vi "RTS Open TDMS Asycronous.vi"(6 "Tree Selection":T1, 7 "Debug":bool, 8 "Error In":errorcluster, 11 "TDMS Data Save Input":T2) -> (0 "Error Out":errorcluster, 3 "TDMS Data Save Output":T2)   [LabVIEW 2016]
uses:
  Type Definitions/RTS TDMS Filename Locations.ctl
  Type Definitions/RTS Room Selector.ctl
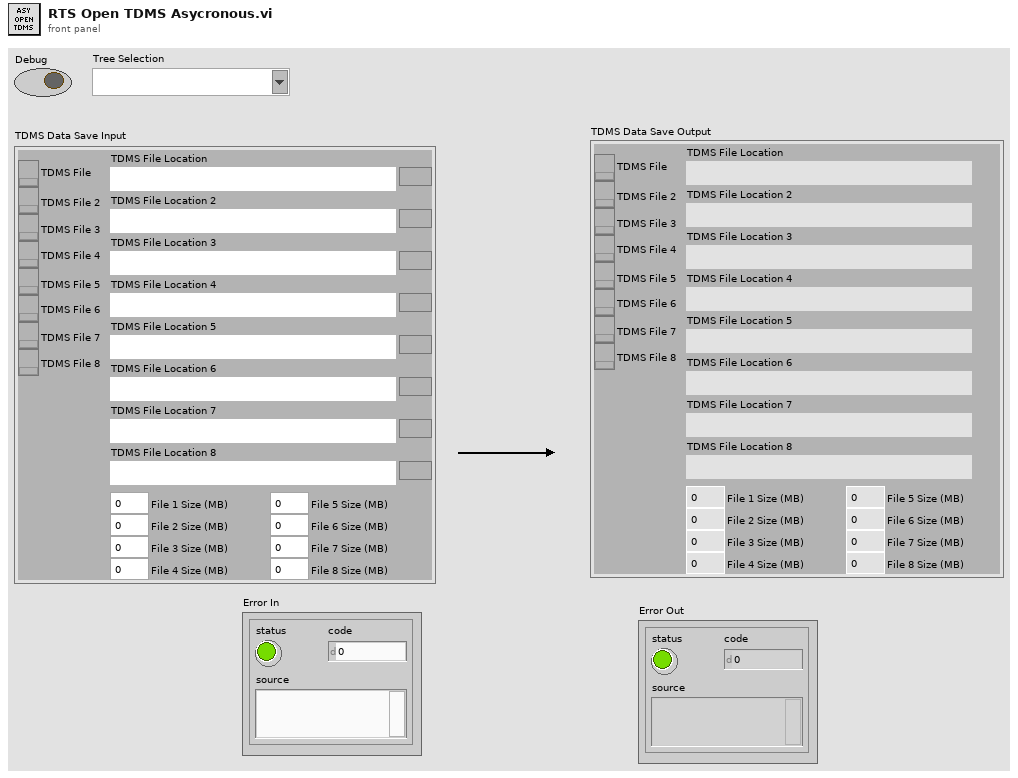
[diagram p1: front panel]
types:
  T1 = typedef "RTS Room Selector.ctl" = string
  T2 = typedef "RTS TDMS Filename Locations.ctl" = cluster{"TDMS File":refnum<k34>, "TDMS File Location":path, "TDMS File Location 2":path, "TDMS File Location 3":path, "TDMS File Location 4":path, "TDMS File Location 5":path, "TDMS File Location 6":path, "TDMS File Location 7":path, "TDMS File Location 8":path, "TDMS File 2":refnum<k34>, "TDMS File 3":refnum<k34>, "TDMS File 4":refnum<k34>, "TDMS File 5":refnum<k34>, "TDMS File 6":refnum<k34>, "TDMS File 7":refnum<k34>, "TDMS File 8":refnum<k34>, "File 1 Size (MB)":dbl, "File 2 Size (MB)":dbl, "File 3 Size (MB)":dbl, "File 4 Size (MB)":dbl, "File 5 Size (MB)":dbl, "File 6 Size (MB)":dbl, "File 7 Size (MB)":dbl, "File 8 Size (MB)":dbl}
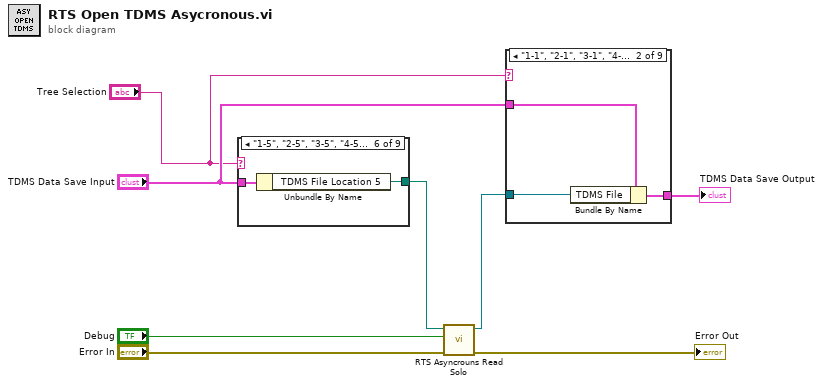
[diagram p0: block diagram]
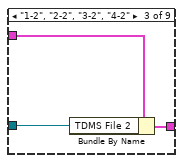
[diagram p3: hidden frame]
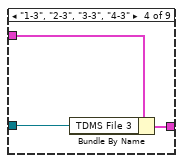
[diagram p4: hidden frame]
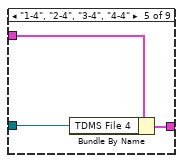
[diagram p5: hidden frame]
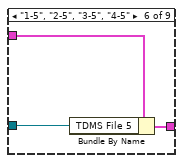
[diagram p6: hidden frame]
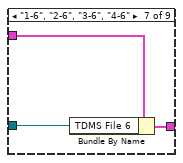
[diagram p7: hidden frame]
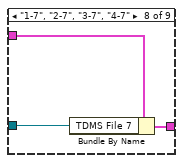
[diagram p8: hidden frame]
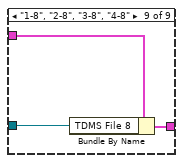
[diagram p9: hidden frame]
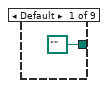
[diagram p10: hidden frame]
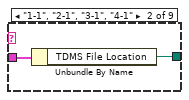
[diagram p11: hidden frame]
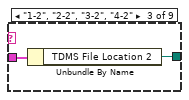
[diagram p12: hidden frame]
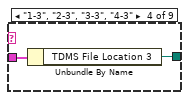
[diagram p13: hidden frame]
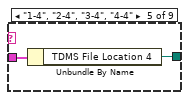
[diagram p14: hidden frame]
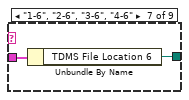
[diagram p15: hidden frame]
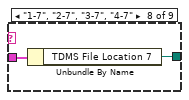
[diagram p16: hidden frame]
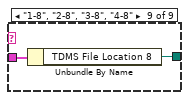
[diagram p17: hidden frame]
diagram:
  n1 = case shown="\"1-5\", \"2-5\", \"3-5\", \"4-5\"" "Tree Selection" {
    tunnel: "TDMS Data Save Input" -> [_ w11 w13 w15 w17 w19 w21 w23 w25]
    tunnel: [path "" ("TDMS File Location 8") w10 w12 w14 w16 w18 w20 w22 w24] -> w6
    frame Default {
    }
    frame "1-1", "2-1", "3-1", "4-1" {
      n2 = Unbundle By Name(w11) -> ("TDMS File Location"=w10:path)
    }
    frame "1-2", "2-2", "3-2", "4-2" {
      n3 = Unbundle By Name(w13) -> ("TDMS File Location 2"=w12:path)
    }
    frame "1-3", "2-3", "3-3", "4-3" {
      n4 = Unbundle By Name(w15) -> ("TDMS File Location 3"=w14:path)
    }
    frame "1-4", "2-4", "3-4", "4-4" {
      n5 = Unbundle By Name(w17) -> ("TDMS File Location 4"=w16:path)
    }
    frame "1-5", "2-5", "3-5", "4-5" {
      n6 = Unbundle By Name(w19) -> ("TDMS File Location 5"=w18:path)
    }
    frame "1-6", "2-6", "3-6", "4-6" {
      n7 = Unbundle By Name(w21) -> ("TDMS File Location 6"=w20:path)
    }
    frame "1-7", "2-7", "3-7", "4-7" {
      n8 = Unbundle By Name(w23) -> ("TDMS File Location 7"=w22:path)
    }
    frame "1-8", "2-8", "3-8", "4-8" {
      n9 = Unbundle By Name(w25) -> ("TDMS File Location 8"=w24:path)
    }
  }
  n10 = call "RTS Asyncrouns Read Solo.vi"("error in (no error)"="Error In", "Debug"="Debug", "TDMS File Location 8"=w6) -> ("error out"=→"Error Out":errorcluster, "Refnum out"=w4:refnum<k34>)  [unwired: 7 in]
  n11 = case shown="\"1-1\", \"2-1\", \"3-1\", \"4-1\"" "Tree Selection" {
    tunnel: "TDMS Data Save Input" -> [w26 w29 w32 w35 w38 w41 w44 w47 w50]
    tunnel: w4 -> [_ w27 w30 w33 w37 w39 w42 w45 w48]
    tunnel: [w26 w28 w31 w34 w36 w40 w43 w46 w49] -> w3
    frame Default {
    }
    frame "1-1", "2-1", "3-1", "4-1" {
      n12 = Bundle By Name(cluster=w29, "TDMS File"=w27) -> (w28:T2)
    }
    frame "1-2", "2-2", "3-2", "4-2" {
      n13 = Bundle By Name(cluster=w32, "TDMS File 2"=w30) -> (w31:T2)
    }
    frame "1-3", "2-3", "3-3", "4-3" {
      n14 = Bundle By Name(cluster=w35, "TDMS File 3"=w33) -> (w34:T2)
    }
    frame "1-4", "2-4", "3-4", "4-4" {
      n15 = Bundle By Name(cluster=w38, "TDMS File 4"=w37) -> (w36:T2)
    }
    frame "1-5", "2-5", "3-5", "4-5" {
      n16 = Bundle By Name(cluster=w41, "TDMS File 5"=w39) -> (w40:T2)
    }
    frame "1-6", "2-6", "3-6", "4-6" {
      n17 = Bundle By Name(cluster=w44, "TDMS File 6"=w42) -> (w43:T2)
    }
    frame "1-7", "2-7", "3-7", "4-7" {
      n18 = Bundle By Name(cluster=w47, "TDMS File 7"=w45) -> (w46:T2)
    }
    frame "1-8", "2-8", "3-8", "4-8" {
      n19 = Bundle By Name(cluster=w50, "TDMS File 8"=w48) -> (w49:T2)
    }
  }
  "TDMS Data Save Output" <- w3
